vi "SENS_CORR_CSET_NAME.vi"(0 "VISA IN":refnum<visa-resource-name>, 1 "Calset Name":string, 5 "error in":errorcluster, 7 "Channel":i32) -> (14 "VISA Out":refnum<visa-resource-name>, 19 "error out":errorcluster)   [LabVIEW 2018, in "PNA-X.lvlib"]
doc: "SENSe<cnum>:CORRection:CSET:NAME <string> \n(Read-Write) Sets or queries the name of the Cal Set currently applied to the specified channel. \nParameters \n<cnum> Any existing channel number. If unspecified, value is set to 1 \n<string> Name of the Cal Set. Spaces or punctuation NOT allowed. \nExamples SENS:CORR:CSET:NAME 'MyCalSet' \nsense2:correction:cset:name 'thisCalSet' \nQuery Syntax SENSe<cnum>:CORRection:CSET:NAME? \nReturn Type String \nDefault Not Applicable"
uses:
  PNA-X.lvlib
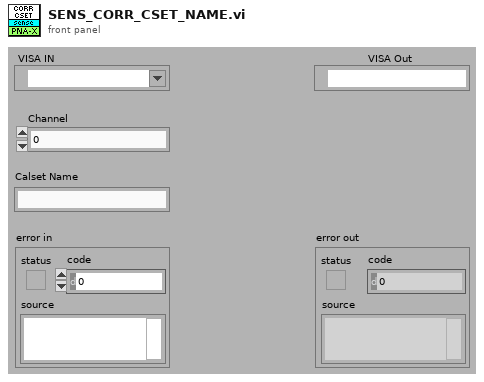
[diagram p1: front panel]
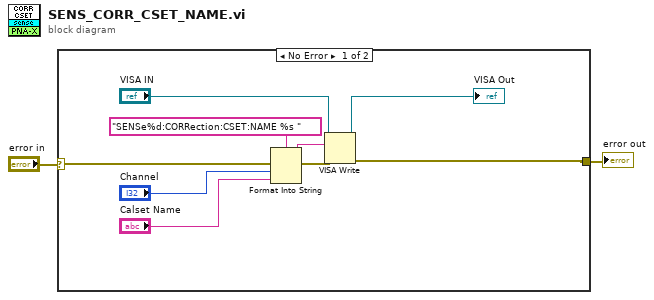
[diagram p0: block diagram]
diagram:
  n1 = case shown="No Error" "error in" {
    selector: "error in" -> [w11 w12]
    tunnel: [w6 w12] -> w1
    frame No Error {
      n2 = Format Into String(format string="SENSe%d:CORRection:CSET:NAME %s " ("Cmdline"), error in=w11, "Channel", "Calset Name") -> (resulting string=w9:string, error out=w10:errorcluster)  [unwired: 1 in]
      n3 = VISA Write(VISA resource name="VISA IN", write buffer=w9, error in (no error)=w10) -> (VISA resource name out=→"VISA Out":refnum<visa-resource-name>, error out=w6:errorcluster)  [unwired: 1 out]
    }
    frame Error {
    }
  }
  "error out" <- w1
